vi "ISO String To Timestamp.vi"(8 "error in (no error)":errorcluster, 11 "ISO Timestamp String":string) -> (0 "error out":errorcluster, 3 "Time Stamp":timestamp)   [LabVIEW 2013, in "JKI JSON Serialization.lvlib" / "JSON Deserializer.lvclass"]
doc: "Converts ISO formatted timestamp string to a LabVIEW timestamp."
uses:
  JSON Deserializer.lvclass
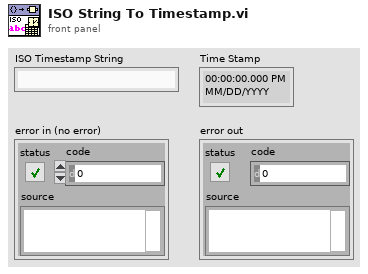
[diagram p1: front panel]
types:
  T1 = typedef "LVDateTimeRec.ctl" = cluster{"fractional second":dbl, "second":i32, "minute":i32, "hour":i32, "day of month":i32, "month":i32, "year":i32, "day of week":i32, "day of year":i32, "DST":i32}
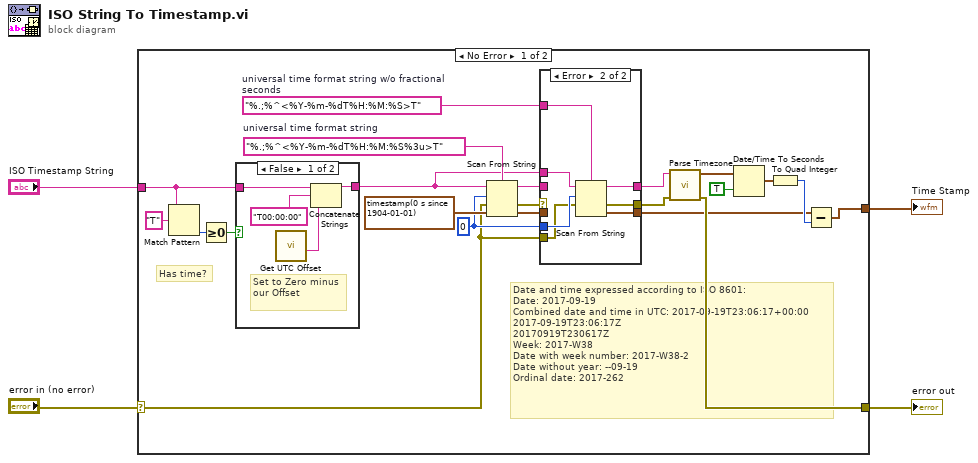
[diagram p0: block diagram]
diagram:
  n1 = case shown="No Error" "error in (no error)" {
    selector: "error in (no error)" -> [w10 w42]
    tunnel: [w26 _] -> w4
    tunnel: [w21 w42] -> w3
    tunnel: "ISO Timestamp String" -> [w7 _]
    frame No Error {
      w12 = "%.;%^<%Y-%m-%dT%H:%M:%S>T"  # universal time format string w/o fractional seconds
      w13 = u32 0 ("initial scan location")
      w19 = "%.;%^<%Y-%m-%dT%H:%M:%S%3u>T"  # universal time format string
      # "Has time?"
      # "Date and time expressed according to ISO 8601:\nDate:\t2017-09-19\nCombined date and time in UTC:\t2017-09-19T23:06:17+00:00\n2017-09-19T23:06:17Z\n20170919T230617Z\nWeek:\t2017-W38\nDate with week number:\t2017-W38-2\nDate without year:\t--09-19\nOrdinal date:\t2017-262"
      n2 = Match Pattern(string=w7, regular expression="T") -> (offset past match=w8:i32)  [unwired: 1 in, 3 out]
      n3 = Greater Or Equal To 0?(x=w8) -> (x >= 0?=w6:bool)
      n4 = case shown="False" w6 {
        tunnel: w7 -> [w30 w31]
        tunnel: [w27 w31] -> w5
        frame False {
          # "Set to Zero minus our Offset"
          n5 = call "Get UTC Offset.vi"() -> ("UTC Offset String"=w28:string)  [unwired: 10 in, 1 out]
          n6 = Concatenate Strings(w30, "T00:00:00" ("string"), w28) -> (w27:string)
        }
        frame True {
        }
      }
      n7 = Scan From String(format string=w19, input string=w5, initial scan location=w13, error in=w10, default 1=timestamp(0 s since 1904-01-01) ("default value 1")) -> (remaining string=w17:string, error out=w18:errorcluster, output 1=w15:timestamp)  [unwired: 1 out]
      n8 = case shown="Error" w18 {
        selector: w18 -> [w33 _]
        tunnel: w17 -> [w34 _]
        tunnel: [w34 w37] -> w16
        tunnel: w15 -> [w32 _]
        tunnel: [w33 w36] -> w14
        tunnel: w10 -> [_ w39]
        tunnel: w5 -> [_ w41]
        tunnel: w13 -> [_ w40]
        tunnel: w12 -> [_ w38]
        tunnel: [w32 w35] -> w11
        frame No Error {
        }
        frame Error {
          n9 = Scan From String(format string=w38, input string=w41, initial scan location=w40, error in=w39) -> (remaining string=w37:string, error out=w36:errorcluster, output 1=w35:timestamp)  [unwired: 1 in, 1 out]
        }
      }
      n10 = call "Parse Timezone.vi"("error in (no error)"=w14, "Timezone String"=w16) -> ("error out"=w21:errorcluster, "time zone offset"=w22:T1)  [unwired: 8 in]
      n11 = Date/Time To Seconds(1:TRUE ("is UTC (F)"), 2:w22) -> (0:w24:timestamp)
      n12 = To Quad Integer(1:w24) -> (0:w25:i64)
      n13 = Subtract(x=w11, y=w25) -> (x-y=w26:timestamp)
    }
    frame Error {
    }
  }
  "Time Stamp" <- w4
  "error out" <- w3
